vi "Home Y Axis.vi"(8 "error in (no error)":errorcluster, 11 "Synchronous Home in":refnum<class "Sync 2-Axis Stage Controller.lvclass">) -> (0 "error out":errorcluster, 3 "Synchronous Home out":refnum<class "Sync 2-Axis Stage Controller.lvclass">)   [LabVIEW 2022 SP3, in "Sync 2-Axis Stage Controller.lvclass"]
uses:
  Sync 2-Axis Stage Controller.lvclass
  Axis Objects/iMotion Controller/iMotion Controller.lvclass
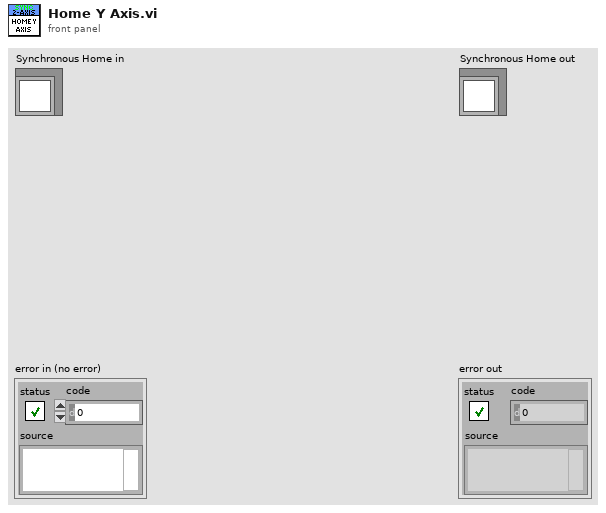
[diagram p1: front panel]
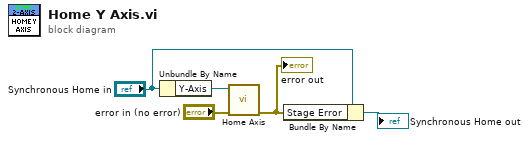
[diagram p0: block diagram]
diagram:
  n1 = Unbundle By Name("Synchronous Home in") -> ("Y-Axis"=w4:refnum<class "iMotion Controller.lvclass">)
  n2 = call-dynamic "Home Axis.vi"("error in (no error)"="error in (no error)", "iMotion Controller in"=w4) -> ("error out"=w1:errorcluster)  [unwired: 8 in, 1 out]
  "error out" <- w1
  n3 = Bundle By Name(cluster="Synchronous Home in", "Stage Error"=w1) -> (→"Synchronous Home out":refnum<class "Sync 2-Axis Stage Controller.lvclass">)
